vi "Add Time to Map.vi"(8 "error in (no error)":errorcluster, 9 "Times":variant, 10 "map in":map{string, map{string, string[]}}(c390), 11 "LV-Data.PGSQL in":refnum<class "LV-Data.PGSQL.lvclass">) -> (0 "error out":errorcluster, 2 "map out":map{string, map{string, string[]}}(c390), 3 "LV-Data.PGSQL out":refnum<class "LV-Data.PGSQL.lvclass">)   [LabVIEW 2019, in "LV-Data.PGSQL.lvclass"]
uses:
  LV-Data.PGSQL.lvclass
  Typedefs/Time.Datatype--enum.ctl
  <vilib>/Utility/Data Type/NI_Data Type.lvlib
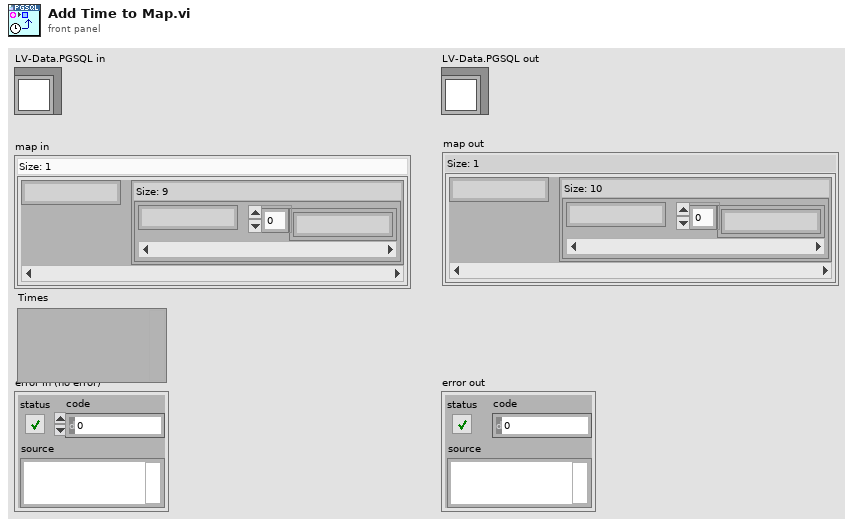
[diagram p1: front panel]
types:
  T1 = typedef "LV-Data.PGSQL.lvclass/Time.Datatype--enum.ctl" = enum16{"timestamp without time zone", "timestamp with time zone"}
  T2 = typedef "NI_Data Type.lvlib/Data Type.ctl" = enum8{"Invalid Type", "Void", "I8", "I16", "I32", "I64", "U8", "U16", "U32", "U64", "Single Float", "Double Float", "Extended Float", "Single Complex", "Double Complex", "Extended Complex", "Enum U8", "Enum U16", "Enum U32", "Enum U64", "Single Float With Unit", "Double Float With Unit", "Extended Float With Unit", "Single Complex with Unit", "Double Complex with Unit", "Extended Complex with Unit", "Boolean", "String", "Path", "Picture", "Tag", "Array", "Cluster", "Variant", "LV Variant", "Waveform", "Timestamp", "Digital Waveform", "Digital Data", "ExpressData", "Refnum", "External Data", "VI", "Poly VI", "LabVIEW Class Instance", "Fixed Point", "Set Collection", "Map Collection"}
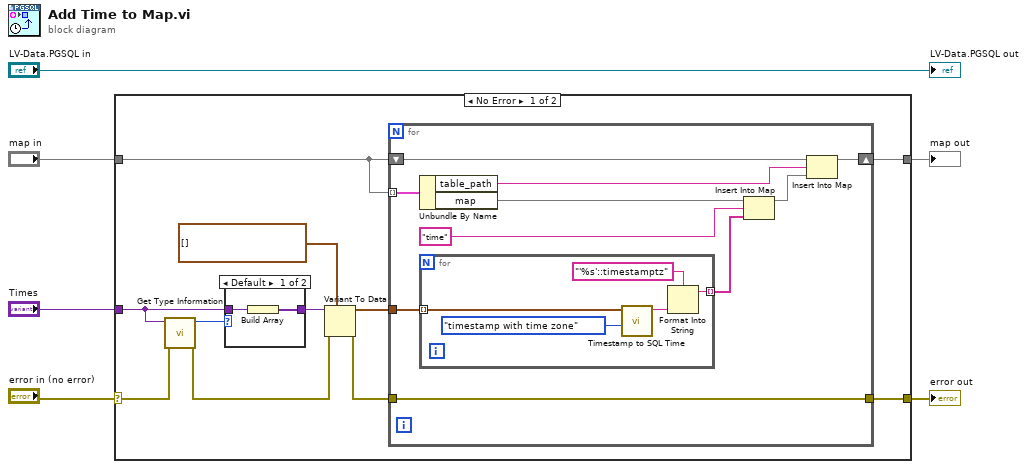
[diagram p0: block diagram]
diagram:
  n1 = case shown="No Error" "error in (no error)" {
    selector: "error in (no error)" -> [w10 w37]
    tunnel: [w17 w36] -> w6
    tunnel: "map in" -> [w16 w36]
    tunnel: [w15 w37] -> w4
    tunnel: "Times" -> [w7 _]
    frame No Error {
      n2 = call <vilib>:"Get Type Information.vi"("error in (no error)"=w10, "variant"=w7) -> ("error out"=w12:errorcluster, "type"=w14:T2)  [unwired: 5 in, 3 out]
      n3 = case shown="Default" w14 {
        tunnel: w7 -> [w19 w20]
        tunnel: [w18 w20] -> w13
        frame Default {
          n4 = Build Array(w19) -> (w18:variant[])
        }
        frame "Array" {
        }
      }
      n5 = Variant To Data(error in=w12, type=timestamp[] [] ("Times"), Variant=w13) -> (data=w11:timestamp[], error out=w9:errorcluster)
      n6 = for {
        tunnel: w11 -> [w27]
        shift-right: [w30] -> w17
        shift-left: w16 -> [w26]
        tunnel: w9 -> [w25]
        tunnel: [w25] -> w15
        tunnel: w16 -> [w23] mode=indexing
        n7 = Unbundle By Name(w23) -> ("table_path"=w21:string, "map"=w22:map{string, string[]})
        n8 = for {
          tunnel: [w33] -> w28 mode=indexing
          tunnel: w27 -> [w32] mode=indexing
          n9 = call "Timestamp to SQL Time.vi"("Time Datatype"=Time.Datatype--enum."timestamp with time zone", "Timestamp"=w32) -> ("date/time string"=w35:string)  [unwired: 9 in]
          n10 = Format Into String(format string="'%s'::timestamptz" ("delimiter (Tab)"), w35) -> (resulting string=w33:string)  [unwired: 2 in, 1 out]
        }
        n11 = Insert Into Map(map in=w22, key="time", value=w28) -> (map out=w29:map{string, string[]})  [unwired: 2 out]
        n12 = Insert Into Map(map in=w26, key=w21, value=w29) -> (map out=w30:map{string, map{string, string[]}})  [unwired: 2 out]
      }
    }
    frame Error {
    }
  }
  "map out" <- w6
  "error out" <- w4
  "LV-Data.PGSQL out" <- "LV-Data.PGSQL in"
